vi "Write data depth.vi"(4 "Error In":errorcluster, 6 "data depth":i32, 7 "Set Data Buffer Depth in":refnum<class "Remote Access Commands_Set Data Buffer Depth.lvclass">) -> (0 "Error Out":errorcluster, 3 "Set Data Buffer Depth out":refnum<class "Remote Access Commands_Set Data Buffer Depth.lvclass">)   [LabVIEW 2015, in "Startup Processes.lvlib" / "Remote Access Commands_Set Data Buffer Depth.lvclass"]
uses:
  Remote Access Commands_Set Data Buffer Depth.lvclass
  Remote Access Commands_Set Data Buffer Depth.lvclass/Remote Access Commands_Set Data Buffer Depth.ctl
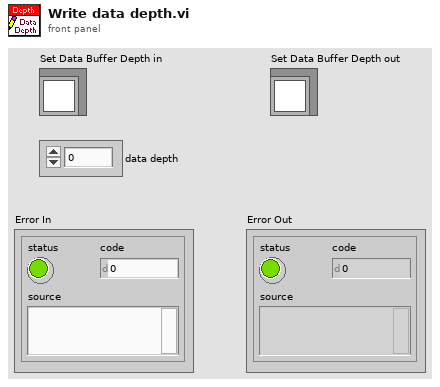
[diagram p1: front panel]
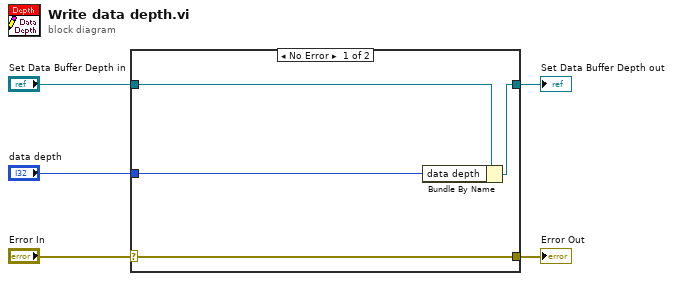
[diagram p0: block diagram]
diagram:
  n1 = case shown="No Error" "Error In" {
    selector: "Error In" -> [w9 w10]
    tunnel: [w9 w10] -> w4
    tunnel: [w7 w11] -> w2
    tunnel: "Set Data Buffer Depth in" -> [w8 w11]
    tunnel: "data depth" -> [w6 _]
    frame No Error {
      n2 = Bundle By Name(cluster=w8, "data depth"=w6) -> (w7:refnum<class "Remote Access Commands_Set Data Buffer Depth.lvclass">)
    }
    frame Error {
    }
  }
  "Error Out" <- w4
  "Set Data Buffer Depth out" <- w2
